vi "SetBooleanFlags.vi"(0 "machine name (\"\":  open local reference)":string="10.0.7.201", 5 "Control Name":string="clear err", 9 "vi path":path=path "C:/g/jma-poc-clean/src/LV-RT-Host/Top-Level/L1 Tester.vi", 11 "error in (no error)":errorcluster) -> (15 "error out":errorcluster)   [LabVIEW 2019]
panel:
  in  "boolean value":bool=TRUE
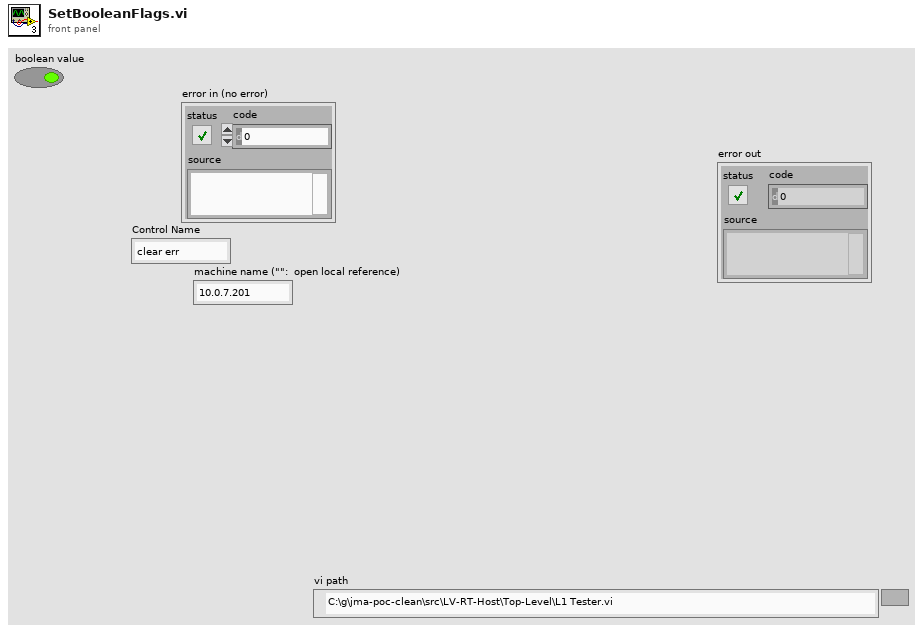
[diagram p1: front panel]
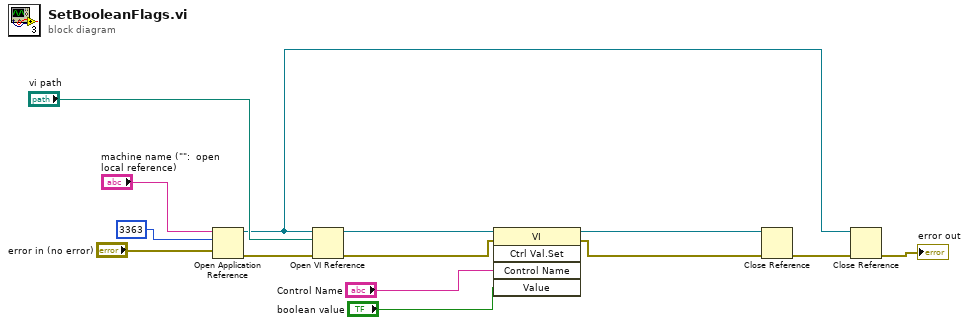
[diagram p0: block diagram]
diagram:
  n1 = Open Application Reference(8:"error in (no error)", 10:u16 3363 ("port number or service name (3363)"), 11:"machine name (\"\":  open local reference)") -> (0:w13:errorcluster, 3:w7:refnum<vi>)  [unwired: 1 in]
  n2 = Open VI Reference(application reference (local)=w7, vi path="vi path", error in (no error)=w13) -> (vi reference=w8:refnum<vi>, error out=w6:errorcluster)  [unwired: 3 in]
  n3 = invoke class="VI" method="Ctrl Val.Set"(reference=w8, error in=w6, "Control Name"="Control Name", "Value"="boolean value") -> (reference out=w3:refnum<vi>, error out=w4:errorcluster)  [unwired: 1 in, 3 out]
  n4 = Close Reference(reference=w3, error in (no error)=w4) -> (error out=w10:errorcluster)
  n5 = Close Reference(reference=w7, error in (no error)=w10) -> (error out=→"error out":errorcluster)
